vi "Configure.vi"(8 "error in":errorcluster, 10 "name":string, 11 "CRDS in":refnum<class "CRDS.lvclass">) -> (0 "error out":errorcluster, 3 "CRDS out":refnum<class "CRDS.lvclass">)   [LabVIEW 2015, in "CRDS.lvclass"]
doc: "Configure the Instrument object. The default behavior is to provide a name and define a command enqueuer."
uses:
  CRDS.lvclass
  Cell/Get Tau Method.ctl
  Instrument/Instrument.lvclass/Instrument.ctl
  CRDS.lvclass/CRDS.ctl
  Cell/CRDS Cell.lvclass/CRDS Cell.ctl
  Cell/Write Data.vi
  Cell/Write Nremove.vi
  Instrument/Read Cfg Session.vi
  <vilib>/Utility/config.llb/Read Key (String).vi
  <vilib>/Utility/config.llb/Read Key (Boolean).vi
  <vilib>/Utility/config.llb/Read Key (Double).vi
  Data/Main/Read CellData.vi
  General/Atmospheric/Atmospheric Constants.vi
  Cell/Write CalType.vi
  Cell/Write errorCalOn.vi
  Cell/Write optTimeConst.vi
  Cell/Write lambda.vi
  Data/Main/Write CellData.vi
  Instrument/Instrument.lvclass
  <userlib>/_Session Fwk/Session - Root.lvclass
  Data/Cell/CRDS Cell Data.lvclass
  Session APIs/File Access/Config Data/Config Data.lvclass
  <vilib>/Utility/config.llb/NI_LVConfig.lvlib
  <vilib>/NI/Tools/String/Tools_String.lvlib
  Data/Main/CRDS Data.lvclass
  Cell/CRDS Cell.lvclass
  General/Atmospheric/Atmospheric Library.lvlib
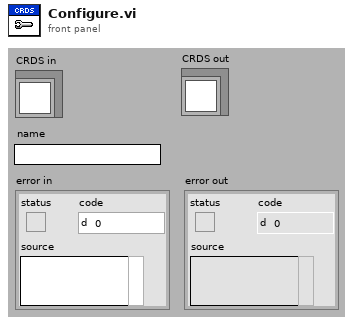
[diagram p1: front panel]
types:
  T1 = typedef "Get Tau Method.ctl" = enum8{"DFT-1", "DFT-5", "LRS"}
  T2 = typedef "Session - Root.lvclass/Session Handle.ctl" = refnum<data-value>
  T3 = typedef "NI_LVConfig.lvlib/Config Data RefNum.ctl" = refnum<k1>
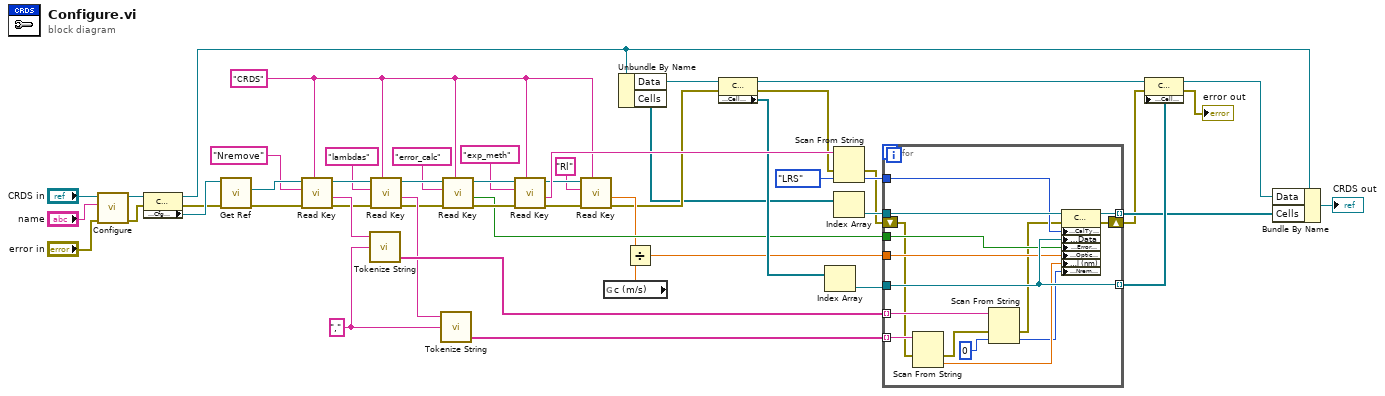
[diagram p0: block diagram]
diagram:
  w40 = "," ("delimiter ([\\s\\t\\n\\r]+)")
  w28 = "CRDS" ("section")
  n1 = call-parent "Configure.vi"("error in"="error in", "name"="name", "Instrument in"="CRDS in") -> ("error out"=w11:errorcluster, "Instrument out"=w9:refnum<class "CRDS.lvclass">)  [unwired: 7 in]
  n2 = property class="CRDS"(reference=w9, error in=w11) -> (reference out=w8:refnum<class "CRDS.lvclass">, error out=w10:errorcluster, "Accessors:Cfg Session"=w49:T2)
  n3 = call "Get Ref.vi"("error in"=w10, "Session Handle In"=w49) -> ("error out"=w7:errorcluster, "Ref"=w48:T3)  [unwired: 7 in, 1 out]
  n4 = call-poly <vilib>:"Read Key.vi"("section"=w28, "error in (no error)"=w7, "key"="Nremove", "refnum"=w48) -> ("error out"=w44:errorcluster, "value"=w46:string, "refnum out"=w45:T3)  [unwired: 4 in, 1 out]
  n5 = call <vilib>:"Tokenize String.vi"("delimiter ([\\s\\t\\n\\r]+)"=w40, "input string"=w46) -> ("token array"=w43:string[])  [unwired: 2 in, 1 out]
  n6 = call-poly <vilib>:"Read Key.vi"("section"=w28, "error in (no error)"=w44, "key"="lambdas", "refnum"=w45) -> ("error out"=w37:errorcluster, "value"=w41:string, "refnum out"=w38:T3)  [unwired: 4 in, 1 out]
  n7 = call <vilib>:"Tokenize String.vi"("delimiter ([\\s\\t\\n\\r]+)"=w40, "input string"=w41) -> ("token array"=w39:string[])  [unwired: 2 in, 1 out]
  n8 = call-poly <vilib>:"Read Key.vi"("section"=w28, "error in (no error)"=w37, "key"="error_calc", "refnum"=w38) -> ("error out"=w34:errorcluster, "value"=w21:bool, "refnum out"=w35:T3)  [unwired: 4 in, 1 out]
  n9 = call-poly <vilib>:"Read Key.vi"("section"=w28, "error in (no error)"=w34, "key"="exp_meth", "refnum"=w35) -> ("error out"=w29:errorcluster, "value"=w32:string, "refnum out"=w30:T3)  [unwired: 4 in, 1 out]
  n10 = call-poly <vilib>:"Read Key.vi"("section"=w28, "error in (no error)"=w29, "key"="Rl", "refnum"=w30) -> ("error out"=w6:errorcluster, "value"=w19:dbl)  [unwired: 4 in, 2 out]
  n11 = global read "Atmospheric Constants.vi" "c (m/s)"() -> (w20:dbl)
  n12 = Unbundle By Name(w8) -> ("Data"=w26:refnum<class "CRDS Data.lvclass">, "Cells"=w3:refnum<class "CRDS Cell.lvclass">[])
  n13 = Divide(x=w19, y=w20) -> (x/y=w18:dbl)
  n14 = property class="CRDS"(reference=w26, error in=w6) -> (reference out=w17:refnum<class "CRDS Data.lvclass">, error out=w5:errorcluster, "Data Access:Cell Data"=w25:refnum<class "CRDS Cell Data.lvclass">[])
  n15 = Index Array(array=w25) -> (element=w24:refnum<class "CRDS Cell Data.lvclass">)  [unwired: 1 in]
  n16 = Scan From String(input string=w32, error in=w5, default 1=Get_Tau_Method."LRS" ("CalType")) -> (error out=w4:errorcluster, output 1=w22:T1)  [unwired: 2 in, 2 out]
  n17 = Index Array(array=w3) -> (element=w23:refnum<class "CRDS Cell.lvclass">)  [unwired: 1 in]
  n18 = for {
    tunnel: w43 -> [w66] mode=indexing
    tunnel: w39 -> [w65] mode=indexing
    tunnel: w24 -> [w62]
    tunnel: w23 -> [w64]
    tunnel: w22 -> [w63]
    tunnel: [w62] -> w16 mode=indexing
    tunnel: w21 -> [w61]
    tunnel: w18 -> [w60]
    tunnel: [w59] -> w14 mode=indexing
    shift-right: [w52] -> w2
    shift-left: w4 -> [w55]
    n19 = Scan From String(input string=w65, error in=w55) -> (error out=w54:errorcluster, output 1=w58:dbl)  [unwired: 3 in, 2 out]
    n20 = Scan From String(input string=w66, error in=w54, default 1=0 ("default value 1")) -> (error out=w53:errorcluster, output 1=w56:i32)  [unwired: 2 in, 2 out]
    n21 = property class="CRDS Cell"(reference=w64, error in=w53, "Data Access:CalType"=w63, "Data Access:Data"=w62, "Data Access:Error Cal On?"=w61, "Data Access:Optical Time Constant"=w60, "Data Access:l (nm)"=w58, "Data Access:Nremove"=w56) -> (reference out=w59:refnum<class "CRDS Cell.lvclass">, error out=w52:errorcluster)
  }
  n22 = property class="CRDS"(reference=w17, error in=w2, "Data Access:Cell Data"=w16) -> (reference out=w1:refnum<class "CRDS Data.lvclass">, error out=→"error out":errorcluster)
  n23 = Bundle By Name(cluster=w8, "Data"=w1, "Cells"=w14) -> (→"CRDS out":refnum<class "CRDS.lvclass">)
